vi "NT Tokenize Path.vi"(11 "Name":string) -> (3 "Array":string[](array[string]))   [LabVIEW 2025]
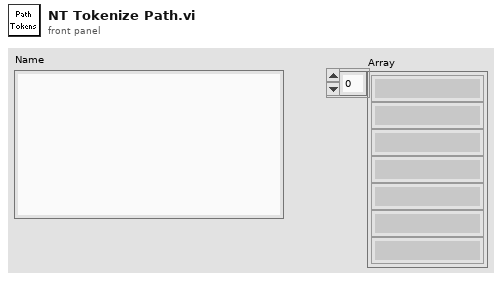
[diagram p1: front panel]
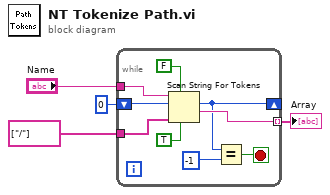
[diagram p0: block diagram]
diagram:
  n1 = while {
    shift-right: [w5] -> _
    shift-left: 0 ("offset past token") -> [w12]
    tunnel: string[] ["/"] ("delimiters (\\s,\\t,\\r,\\n)") -> [w13]
    tunnel: "Name" -> [w9]
    tunnel: [w8] -> w1 mode=indexing
    stop <- w6 stop-if-true
    n2 = Scan String For Tokens(4:TRUE ("use cached delim/oper data? (F)"), 5:FALSE ("use cached delim/oper data? (F)"), 6:w13, 8:w12, 9:w9) -> (1:w8:string, 2:w5:i32)  [unwired: 1 in, 2 out]
    n3 = Equal?(x=w5, y=-1 ("offset past token")) -> (x = y?=w6:bool)
  }
  "Array" <- w1
